vi "Add Headers.vi"(0 "client handle":T2, 1 "BlueLogParent in":refnum<class "BlueLogParent_OpenSource.lvclass">, 5 "HTTP Headers":T1[](array[typedef]), 11 "error IO":errorcluster) -> (4 "client handle":T2, 15 "error IO":errorcluster)   [LabVIEW 2020, in "Blue Easy HTTP OpenSource.lvlib"]
uses:
  Blue Easy HTTP OpenSource.lvlib
  <vilib>/httpClient/ClientHandle.ctl
  HTTP Header.ctl
  <userlib>/Blue Origin/BlueLogParent_OpenSource/BlueLogParentClass/BlueLogParent_OpenSource.lvclass
  <vilib>/httpClient/LabVIEWHTTPClient.lvlib
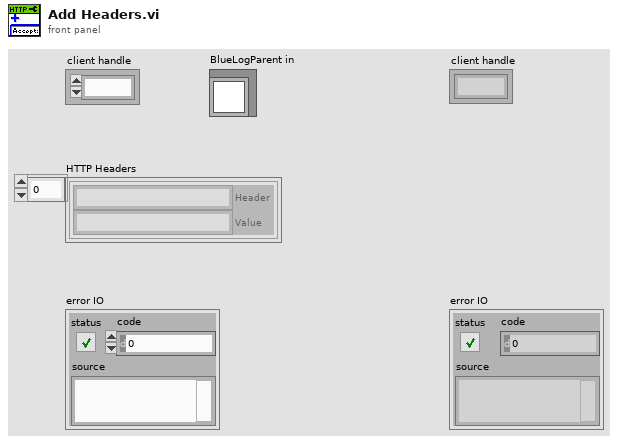
[diagram p1: front panel]
types:
  T1 = typedef "Blue Easy HTTP OpenSource.lvlib/HTTP Header.ctl" = cluster{"Header":string, "Value":string}
  T2 = typedef "LabVIEWHTTPClient.lvlib/ClientHandle.ctl" = refnum<k1>
  T3 = typedef "BlueLogParent_OpenSource.lvclass/BlueLogParentLevel.ctl" = enum16{"DEBUG", "INFO", "WARNING", "ERROR", "CRITICAL"}
  T4 = typedef "BlueLogParent_OpenSource.lvclass/BlueLogParentOptions.ctl" = cluster{"timestamp (now)":dbl, "Call chain (here)":string, "Count (1)":u16, "Font (override)":T5, "Add row separator? (T)":bool}
  T5 = typedef "BlueLogParent_OpenSource.lvclass/BlueLogParentFont.ctl" = cluster{"Font Name":string, "Size":u16, "Bold":bool, "Italic":bool, "Underline":bool, "Strikeout":bool, "Color":u32}
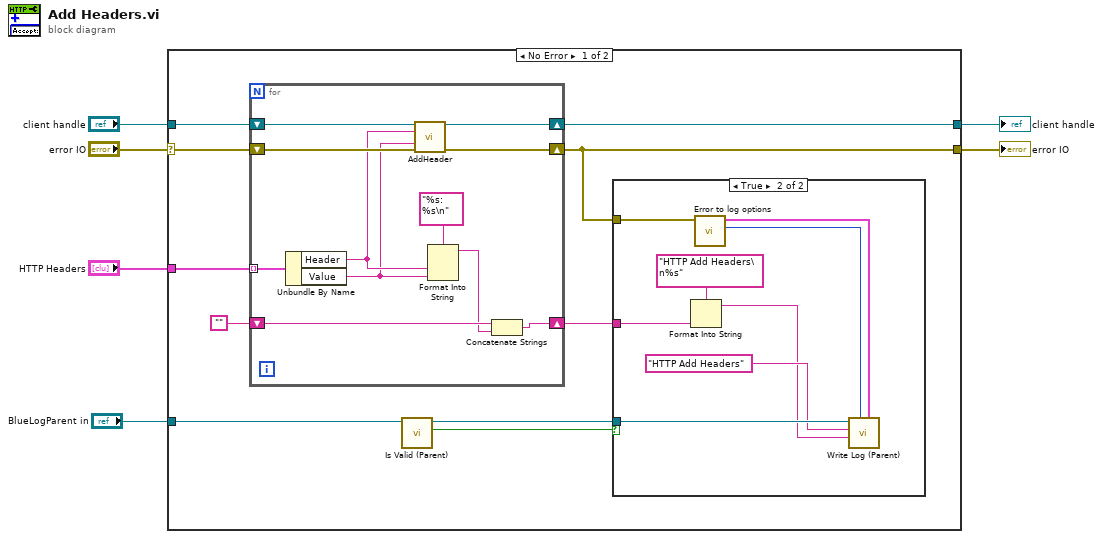
[diagram p0: block diagram]
diagram:
  n1 = case shown="No Error" "error IO" {
    selector: "error IO" -> [w16 w37]
    tunnel: [w15 w37] -> w4
    tunnel: "client handle" -> [w13 w36]
    tunnel: [w14 w36] -> w5
    tunnel: "HTTP Headers" -> [w12 _]
    tunnel: "BlueLogParent in" -> [w7 _]
    frame No Error {
      n2 = for {
        shift-right: [w26] -> w15
        shift-left: w16 -> [w27]
        shift-right: [w25] -> w14
        shift-left: w13 -> [w24]
        tunnel: w12 -> [w23] mode=indexing
        shift-right: [w17] -> w10
        shift-left: "" -> [w19]
        n3 = Unbundle By Name(w23) -> ("Header"=w21:string, "Value"=w20:string)
        n4 = call <vilib>:"AddHeader.vi"("client handle"=w24, "header"=w21, "value"=w20, "error in (no error)"=w27) -> ("client handle out"=w25:T2, "error out"=w26:errorcluster)  [unwired: 10 in]
        n5 = Format Into String(format string="%s: %s\n", w21, w20) -> (resulting string=w18:string)  [unwired: 2 in, 1 out]
        n6 = Concatenate Strings(w19, w18) -> (w17:string)
      }
      n7 = call-dynamic "Is Valid (Parent).vi"("BlueLogParent in"=w7) -> ("Is Valid?"=w8:bool, "BlueLogParent out"=w9:refnum<class "BlueLogParent_OpenSource.lvclass">)  [unwired: 8 in, 1 out]
      n8 = case shown="True" w8 {
        tunnel: w9 -> [_ w33]
        tunnel: w15 -> [_ w30]
        tunnel: w10 -> [_ w34]
        frame False {
        }
        frame True {
          n9 = Format Into String(format string="HTTP Add Headers\n%s", w34) -> (resulting string=w31:string)  [unwired: 2 in, 1 out]
          n10 = call "Error to log options.vi"("error in (no error)"=w30) -> ("Logging level"=w29:T3, "Options"=w28:T4)  [unwired: 9 in]
          n11 = call-dynamic "Write Log (Parent).vi"("Options"=w28, "Logging level (INFO)"=w29, "Message"=w31, "Message Title"="HTTP Add Headers" ("Unique ID"), "BlueLogParent in"=w33) -> ()  [unwired: 5 in, 2 out]
        }
      }
    }
    frame Error {
    }
  }
  "client handle" <- w5
  "error IO" <- w4
